vi "WPI_CameraSend Images To PC Loop.vi"(8 "error in (no error)":errorcluster, 9 "port":u16=1181, 10 "IP CGI string":string="/axis-cgi/mjpg/video.cgi") -> ()   [LabVIEW 2018]
doc: "This VI is used to serve images from one or more named cameras on your robot to the dashboard, SmartDashboard, or compatible web browser. Camera name and type info is published using network tables. Connections are on port 1181 by default and the URL for streaming can be found by looking at the network \"camera\"/streams variable. Cameras that are opened and stored in the name registry are automatically published by that name.\n\nThis VI runs in parallel with other code and should be placed in Robot Main or in Periodic Tasks.\n\nThis software is licensed. Open the labview\\readme\\WPI Robotics Library Open Source License.txt file for more information."
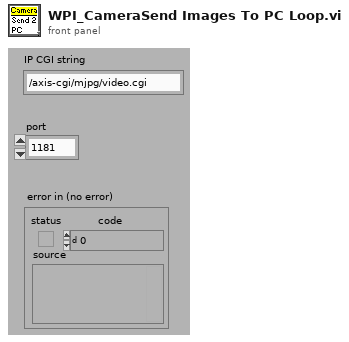
[diagram p1: front panel]
types:
  T1 = enum16{"Standard", "Buffered", "CRLF", "Immediate"}
  T2 = cluster{"token string":string, "token string 2":string}[]
  T3 = cluster{"Type":u32, "Version":u32, "Flags":u32, "SerialNumberHigh":u32, "SerialNumberLow":u32, "BusType":u32, "InterfaceName":string, "VendorName":string, "ModelName":string, "CameraFileName":string, "CameraAttributeURL":string}[]
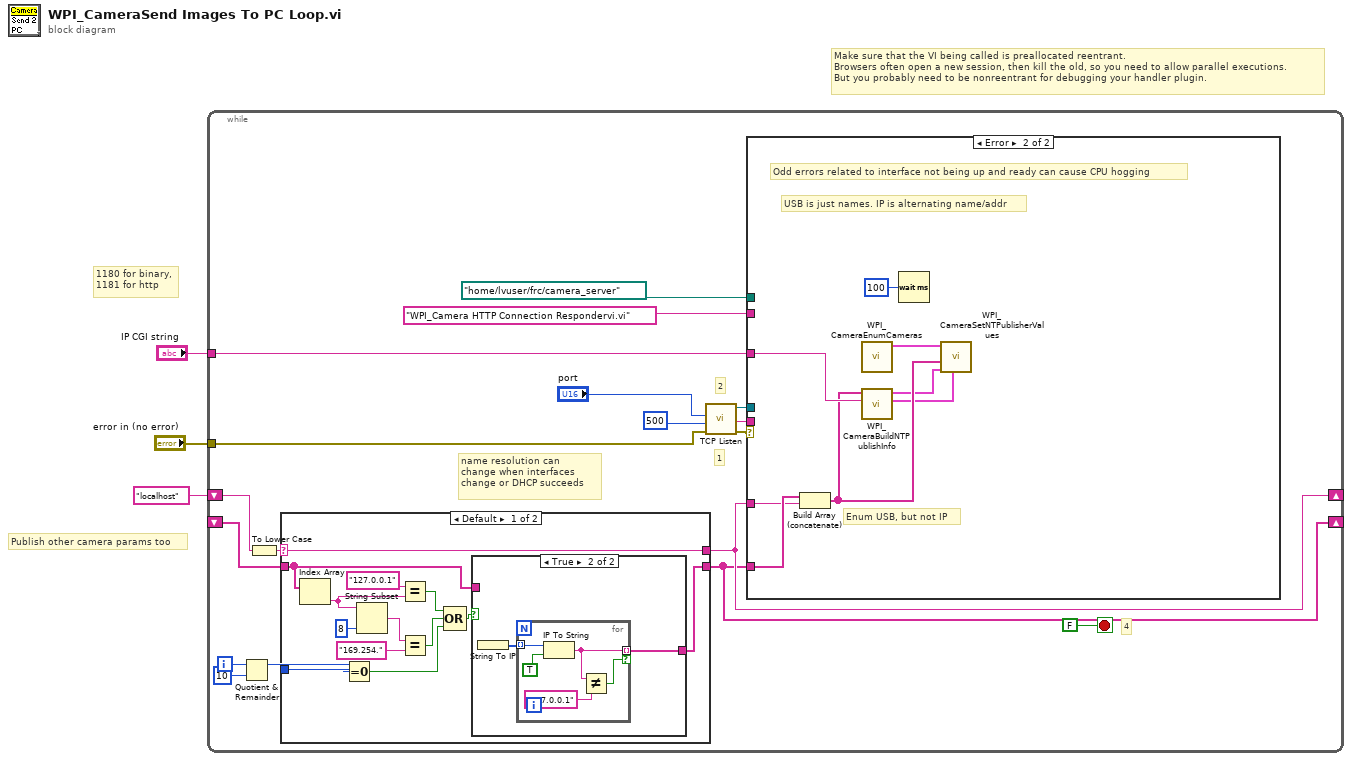
[diagram p0: block diagram]
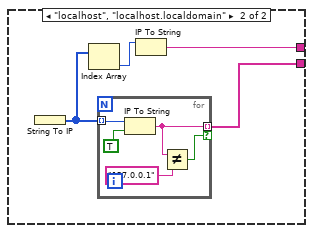
[diagram p3: hidden frame]
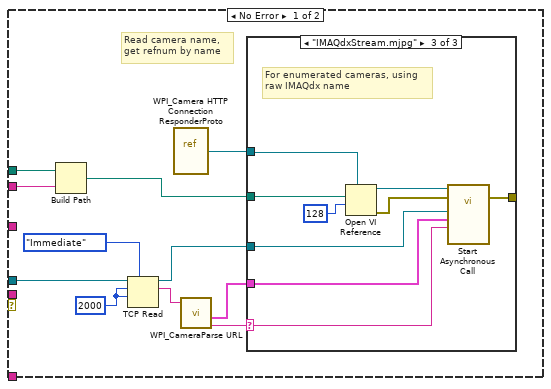
[diagram p4: hidden frame]
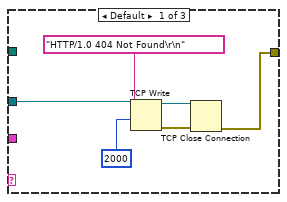
[diagram p5: hidden frame]
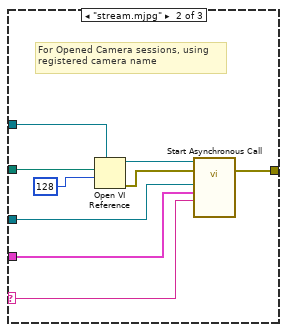
[diagram p6: hidden frame]
diagram:
  # "Make sure that the VI being called is preallocated reentrant.\nBrowsers often open a new session, then kill the old, so you need to allow parallel executions.\nBut you probably need to be nonreentrant for debugging your handler plugin."
  # "Publish other camera params too"
  # "1180 for binary,\n1181 for http"
  n1 = while {
    tunnel: "error in (no error)" -> [w20]
    shift-right: [w12] -> _
    shift-left: "localhost" -> [w13]
    shift-right: [w10] -> _
    shift-left: _ -> [w11]
    tunnel: "IP CGI string" -> [w9]
    i -> [w6]
    stop <- FALSE ("status") stop-if-true
    # "name resolution can\nchange when interfaces\nchange or DHCP succeeds"
    # "4"
    # "1"
    # "2"
    n2 = Quotient & Remainder(x=w6, y=10) -> (x-y*floor(x/y)=w4:i32)  [unwired: 1 out]
    n3 = To Lower Case(string=w13) -> (all lower case string=w14:string)
    n4 = case shown="Default" w14 {
      selector: w14 -> [w34 _]
      tunnel: [w34 w46] -> w12
      tunnel: w11 -> [w23 _]
      tunnel: [w24 w45] -> w10
      tunnel: w4 -> [w26 _]
      frame Default {
        n5 = Index Array(array=w23) -> (element=w22:string)  [unwired: 1 in]
        n6 = Equal To 0?(x=w26) -> (x = 0?=w25:bool)
        n7 = String Subset(string=w22, length (rest)=8 ("length (rest)")) -> (substring=w30:string)  [unwired: 1 in]
        n8 = Equal?(x="127.0.0.1", y=w22) -> (x = y?=w28:bool)
        n9 = Equal?(x=w30, y="169.254.") -> (x = y?=w27:bool)
        n10 = Compound Arithmetic op=OR(w28, w27, w25) -> (w31:bool)
        n11 = case shown="True" w31 {
          tunnel: w23 -> [w35 _]
          tunnel: [w35 w36] -> w24
          frame False {
          }
          frame True {
            n12 = String To IP() -> (0:w37:u32[])  [unwired: 1 in]
            n13 = for {
              tunnel: w37 -> [w41] mode=indexing
              tunnel: [w39] -> w36 mode=indexing if=w38
              n14 = IP To String(1:TRUE ("dot notation? (F)"), 2:w41) -> (0:w39:string)
              n15 = Not Equal?(x=w39, y="127.0.0.1") -> (x != y?=w38:bool)
            }
          }
        }
      }
      frame "localhost", "localhost.localdomain" {
        n16 = String To IP() -> (0:w44:u32[])  [unwired: 1 in]
        n17 = Index Array(array=w44) -> (element=w43:u32)  [unwired: 1 in]
        n18 = for {
          tunnel: w44 -> [w50] mode=indexing
          tunnel: [w48] -> w45 mode=indexing if=w47
          n19 = IP To String(1:TRUE ("dot notation? (F)"), 2:w50) -> (0:w48:string)
          n20 = Not Equal?(x=w48, y="127.0.0.1") -> (x != y?=w47:bool)
        }
        n21 = IP To String(2:w43) -> (0:w46:string)  [unwired: 1 in]
      }
    }
    n22 = call <vilib>:"TCP Listen.vi"("error in (no error)"=w20, "timeout ms (wait forever: -1)"=u16 500 ("port"), "port"="port") -> ("error out"=w17:errorcluster, "remote address"=w21:string, "connection ID"=w19:refnum<k5>)  [unwired: 1 in, 5 out]
    n23 = case shown="Error" w17 {
      tunnel: w21 -> [_ _]
      tunnel: w19 -> [w60 _]
      tunnel: w12 -> [_ w92]
      tunnel: w10 -> [_ w93]
      tunnel: w9 -> [_ w91]
      tunnel: "WPI_Camera HTTP Connection Respondervi.vi" -> [w55 _]
      tunnel: path "/home/lvuser/frc/camera_server" -> [w54 _]
      frame No Error {
        w61 = 2000
        # "Read camera name,\nget refnum by name"
        n24 = Build Path(base path=w54, name or relative path=w55) -> (appended path=w53:path)
        n25 = TCP Read(connection ID=w60, bytes to read=w61, 7:T1."Immediate" ("mode (standard)"), 9:w61) -> (connection ID out=w59:refnum<k5>, data out=w57:string)  [unwired: 1 in, 1 out]
        n26 = vi-ref <vilib>:"WPI_Camera HTTP Connection ResponderProto.vi"() -> (w52:refnum<vi>)
        n27 = call <vilib>:"WPI_CameraParse URL.vi"("URL"=w57) -> ("cgi string"=w56:string, "parameters"=w58:T2)  [unwired: 7 in, 2 out]
        n28 = case shown="\"IMAQdxStream.mjpg\"" w56 {
          selector: w56 -> [_ w70 w79]
          tunnel: w53 -> [_ w77 w86]
          tunnel: w59 -> [w68 w75 w84]
          tunnel: [w63 w73 w82] -> _
          tunnel: w58 -> [_ w72 w81]
          tunnel: w52 -> [_ w69 w78]
          frame Default {
            n29 = TCP Write(connection ID=w68, data in="HTTP/1.0 404 Not Found\r\n" ("regular expression"), 9:2000) -> (connection ID out=w67:refnum<k5>, error out=w64:errorcluster)  [unwired: 1 in, 1 out]
            n30 = TCP Close Connection(connection ID=w67, error in (no error)=w64) -> (error out=w63:errorcluster)  [unwired: 2 out]
          }
          frame "stream.mjpg" {
            # "For Opened Camera sessions, using\nregistered camera name"
            n31 = Open VI Reference(type specifier VI Refnum (for type only)=w69, vi path=w77, options=128) -> (vi reference=w71:refnum<vi>, error out=w74:errorcluster)  [unwired: 3 in]
            n32 = call-by-ref "Start Asynchronous Call"(reference=w71, error in=w74, "CGI String"=w70, "parameters"=w72, "connection ID"=w75) -> (error out=w73:errorcluster)  [unwired: 9 in, 1 out]
          }
          frame "IMAQdxStream.mjpg" {
            # "For enumerated cameras, using\nraw IMAQdx name"
            n33 = Open VI Reference(type specifier VI Refnum (for type only)=w78, vi path=w86, options=128) -> (vi reference=w80:refnum<vi>, error out=w83:errorcluster)  [unwired: 3 in]
            n34 = call-by-ref "Start Asynchronous Call"(reference=w80, error in=w83, "CGI String"=w79, "parameters"=w81, "connection ID"=w84) -> (error out=w82:errorcluster)  [unwired: 9 in, 1 out]
          }
        }
      }
      frame Error {
        # "Enum USB, but not IP"
        # "USB is just names. IP is alternating name/addr"
        # "Odd errors related to interface not being up and ready can cause CPU hogging"
        n35 = Build Array (concatenate)(w93, w92) -> (w89:string[])
        n36 = call <vilib>:"WPI_CameraEnumCameras.vi"() -> ("USB Cams"=w90:T3)  [unwired: 10 in, 1 out]
        n37 = call <vilib>:"WPI_CameraBuildNTPublishInfo.vi"("IP CGI string"=w91, "RIO Addresses"=w89) -> ("Streams"=w87:cluster{string, "URLs":string[]}[], "Sources"=w88:cluster{string, string}[])  [unwired: 8 in]
        n38 = Wait (ms)(milliseconds to wait=u32 100) -> ()  [unwired: 1 out]
        n39 = call <vilib>:"WPI_CameraSetNTPublisherValues.vi"("Streams"=w87, "Sources"=w88, "roboRIO Addresses"=w89, "USB Cams"=w90) -> ()  [unwired: 8 in]
      }
    }
  }
